vi "Add Module to Map.vi"(4 "is Dependency?":bool, 5 "Parent Path":string, 7 "App Ref":refnum<vi>, 9 "Module Type":T1, 10 "Tree Map in":T2, 11 "Library in":refnum<vi>) -> (2 "Tree Map out":T2, 3 "Name":string)   [LabVIEW 2019, in "Panther Dashboard.lvlib"]
uses:
  Panther Dashboard.lvlib
  <vilib>/National Instruments/Tree Map/Tree Map Data.ctl
  Module type--enum.ctl
  Map Attribute--enum.ctl
  <vilib>/National Instruments/Tree Map/Tree Map.lvlib
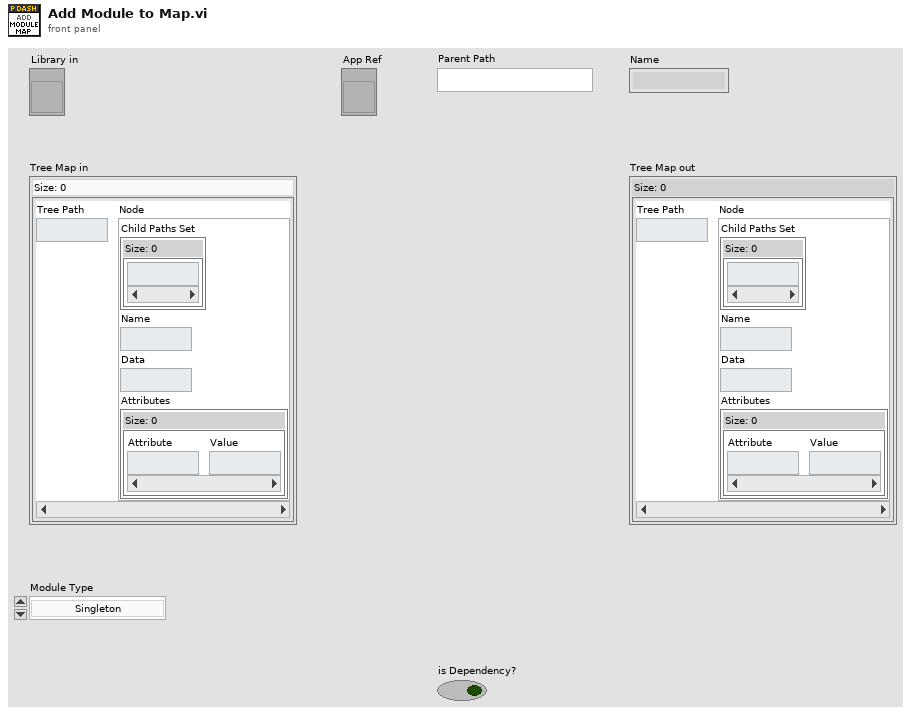
[diagram p1: front panel]
types:
  T1 = typedef "Panther Dashboard.lvlib/Module type--enum.ctl" = enum16{"Singleton", "Cloneable"}
  T2 = typedef "Tree Map.lvlib/Tree Map Data.ctl" = map{string, cluster{"Child Paths Set":set{string}, "Name":string, "Data":string, "Attributes":map{string, string}}}
  T3 = typedef "Panther Dashboard.lvlib/Map Attribute--enum.ctl" = enum16{"Path", "ModuleType", "Module Description", "Dependency?", "Target"}
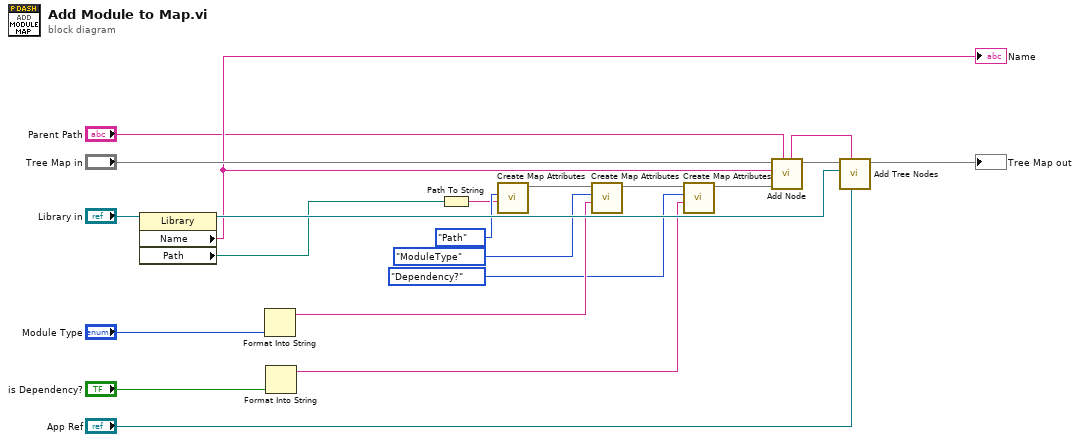
[diagram p0: block diagram]
diagram:
  n1 = property class="Library"(reference="Library in") -> (reference out=w21:refnum<vi>, "Name"=w14:string, "Path"=w5:path)  [unwired: 1 in, 1 out]
  "Name" <- w14
  n2 = Format Into String("Module Type") -> (resulting string=w7:string)  [unwired: 3 in, 1 out]
  n3 = Format Into String("is Dependency?") -> (resulting string=w1:string)  [unwired: 3 in, 1 out]
  n4 = Path To String(path=w5) -> (string=w6:string)
  n5 = call "Create Map Attributes.vi"("Attribute"=w6, "Map Attribute"=Map_Attribute--enum."Path") -> ("Root Attributes"=w10:map{string, string})  [unwired: 9 in]
  n6 = call "Create Map Attributes.vi"("Attribute"=w7, "Map Attribute"=Map_Attribute--enum."ModuleType", "Root Attributes In"=w10) -> ("Root Attributes"=w9:map{string, string})  [unwired: 8 in]
  n7 = call "Create Map Attributes.vi"("Attribute"=w1, "Map Attribute"=Map_Attribute--enum."Dependency?", "Root Attributes In"=w9) -> ("Root Attributes"=w4:map{string, string})  [unwired: 8 in]
  n8 = call <vilib>:"Add Node.vi"("Parent Path"="Parent Path", "Attributes"=w4, "New Node Name"=w14, "Tree Map In"="Tree Map in") -> ("Tree Map Out"=w16:T2, "New Node Path"=w20:string)  [unwired: 5 in, 1 out]
  n9 = call "Add Tree Nodes.vi"("App Ref"="App Ref", "Root path"=w20, "DQMH Lib In"=w21, "Tree Map in"=w16) -> ("Tree Map out"=→"Tree Map out":T2)  [unwired: 7 in]
